vi "Write Source PDF File [ ].vi"(0 "PDF Report IN":refnum<class "PDF Report Class.lvclass">=refnum, 2 "TOC page":cluster{"Start":i32, "Number":i32}, 11 "error in (no error)":errorcluster, 13 "Last PageNumber":i32) -> (4 "PDF Report OUT":refnum<class "PDF Report Class.lvclass">, 15 "error out":errorcluster)   [LabVIEW 2020, in "Exaprom PDF.lvlib"]
doc: "Version 2.0\nDeveloped by Jean-Marc Simard\nCopyright © 2012, Exaprom Inc.\nAll rights reserved.\nLicense: BSD\n\nWith iTextSharp 4.1.6 (http://itextsharp.sourceforge.net)\nunder Mozilla Public License Version 1.1\n(http://www.mozilla.org/MPL/MPL-1.1.html)"
uses:
  <userlib>/labview-PDF-writer-master/Exaprom PDF.lvlib
  <userlib>/labview-PDF-writer-master/LV Class/PDF Report Class/PDF Report Class.lvclass
  <userlib>/labview-PDF-writer-master/LV Class/Fonts Class/Font Class.lvclass
  <userlib>/labview-PDF-writer-master/LV Class/Header and Footer Class/Header and Footer Class.lvclass
  <userlib>/labview-PDF-writer-master/Controls/Concatenate Controls/PDF File and position.ctl
  <userlib>/labview-PDF-writer-master/Controls/Concatenate Controls/PDF file source.ctl
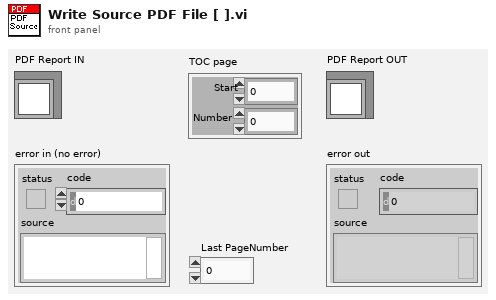
[diagram p1: front panel]
types:
  T1 = typedef "Exaprom PDF.lvlib/PDF File and position.ctl" = cluster{"Path":path, "Pages":string, "Source":T2, "Start at page old":i32, "Start at page new":i32, "Owner password":string}
  T2 = typedef "Exaprom PDF.lvlib/PDF file source.ctl" = enum16{"PDF Report", "File to add"}
  T3 = typedef "Exaprom PDF.lvlib/File Permission Parameters.ctl" = cluster{"User Password":string, "Owner Password":string, "Printing":enum16{"Allow Printing", "Allow Degraded Printing", "Don't Allow Printing"}, "Allow Modify Contents":bool, "Allow Copy":bool, "Allow Modify Annotations":bool, "Allow Fill In ":bool, "Allow Screen Readers":bool, "Allow Assembly":bool}
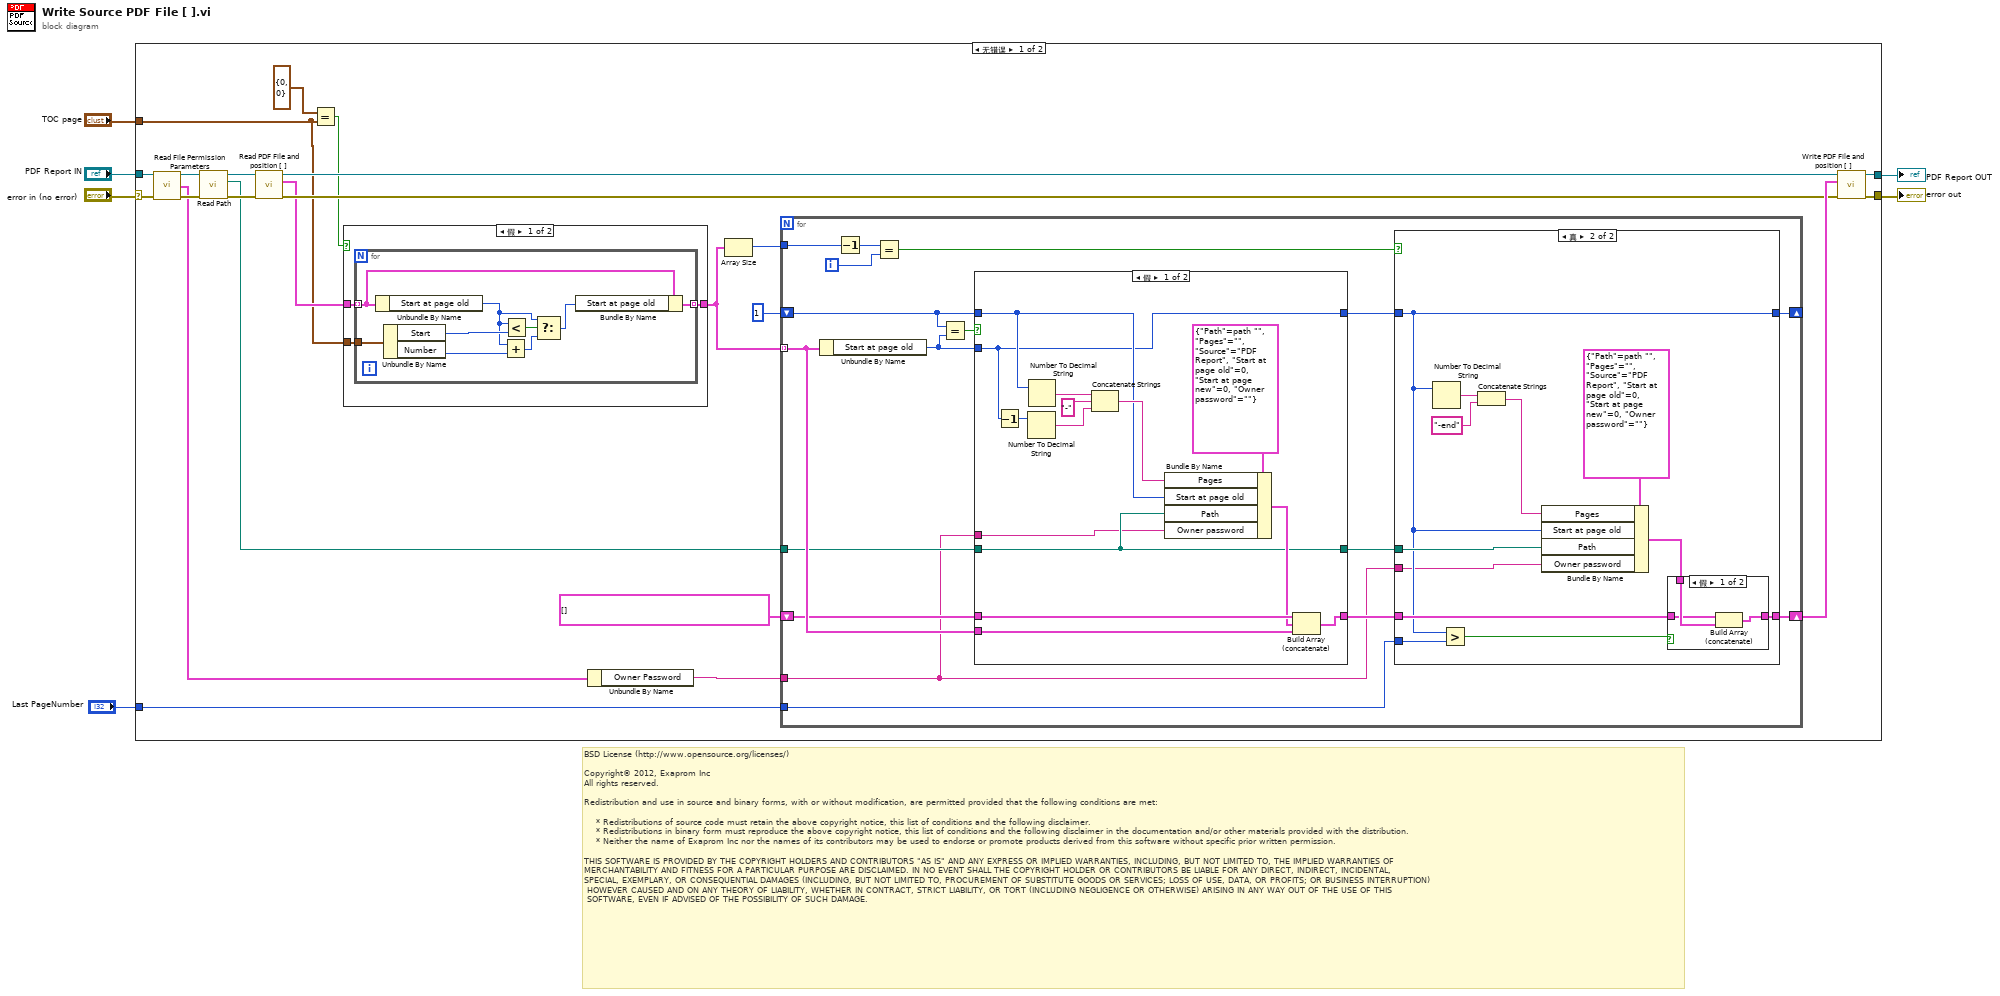
[diagram p0: block diagram]
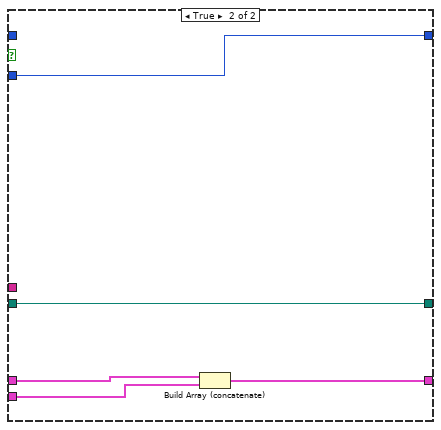
[diagram p5: hidden frame]
diagram:
  # "BSD License (http://www.opensource.org/licenses/)\n\nCopyright© 2012, Exaprom Inc\nAll rights reserved.\n\nRedistribution and use in source and binary forms, with or without modification, are permitted provided that the following conditions are met:\n\n    * Redistributions of source code must retain the above copyright notice, this list of conditions and the following disclaimer.\n    * Redistributions in binary form must reproduce the above copyright notice, this list of conditions and the following disclaimer in the documentation and/or other materials provided with the distribution.\n    * Neither the name of Exaprom Inc nor the names of its contributors may be used to endorse or promote products derived from this software without specific prior written permission.\n\nTHIS SOFTWARE IS PROVIDED BY THE COPYRIGHT HOLDERS AND CONTRIBUTORS \"AS IS\" AND ANY EXPRESS OR IMPLIED WARRANTIES, INCLUDING, BUT NOT LIMITED TO, THE IMPLIED WARRANTIES OF \nMERCHANTABILITY AND FITNESS FOR A PARTICULAR PURPOSE ARE DISCLAIMED. IN NO EVENT SHALL THE COPYRIGHT HOLDER OR CONTRIBUTORS BE LIABLE FOR ANY DIRECT, INDIRECT, INCIDENTAL,\nSPECIAL, EXEMPLARY, OR CONSEQUENTIAL DAMAGES (INCLUDING, BUT NOT LIMITED TO, PROCUREMENT OF SUBSTITUTE GOODS OR SERVICES; LOSS OF USE, DATA, OR PROFITS; OR BUSINESS INTERRUPTION)\n HOWEVER CAUSED AND ON ANY THEORY OF LIABILITY, WHETHER IN CONTRACT, STRICT LIABILITY, OR TORT (INCLUDING NEGLIGENCE OR OTHERWISE) ARISING IN ANY WAY OUT OF THE USE OF THIS\n SOFTWARE, EVEN IF ADVISED OF THE POSSIBILITY OF SUCH DAMAGE."
  n1 = case shown="无错误" "error in (no error)" {
    selector: "error in (no error)" -> [w15 w98]
    tunnel: "PDF Report IN" -> [w18 w97]
    tunnel: [w25 w97] -> w5
    tunnel: [w26 w98] -> w4
    tunnel: "Last PageNumber" -> [w17 _]
    tunnel: "TOC page" -> [w8 _]
    frame No Error {
      n2 = call-dynamic "Read File Permission Parameters.vi"("PDF Report Class in"=w18, "error in (no error)"=w15) -> ("PDF Report Class out"=w16:refnum<class "PDF Report Class.lvclass">, "File Permission Parameters"=w13:T3, "error out"=w14:errorcluster)  [unwired: 11 in]
      n3 = call-dynamic "Read Path.vi"("error in (no error)"=w14, "PDF Report Class in"=w16) -> ("error out"=w21:errorcluster, "Path"=w20:path, "PDF Report Class out"=w19:refnum<class "PDF Report Class.lvclass">)  [unwired: 7 in]
      n4 = call-dynamic "Read PDF File and position [ ].vi"("error in (no error)"=w21, "PDF Report Class in"=w19) -> ("error out"=w23:errorcluster, "PDF File and position [ ]"=w10:T1[], "PDF Report Class out"=w22:refnum<class "PDF Report Class.lvclass">)  [unwired: 7 in]
      n5 = Equal?(x=cluster{"Start":i32, "Number":i32} {"Start"=0, "Number"=0}, y=w8) -> (x = y?=w7:bool)
      n6 = case shown="假" w7 {
        tunnel: w10 -> [w32 w42]
        tunnel: [w31 w42] -> w9
        tunnel: w8 -> [w30 _]
        frame False {
          n7 = for {
            tunnel: w32 -> [w41] mode=indexing
            tunnel: [w40] -> w31 mode=indexing
            tunnel: w30 -> [w39]
            n8 = Unbundle By Name(w41) -> ("Start at page old"=w34:i32)
            n9 = Unbundle By Name(w39) -> ("Start"=w38:i32, "Number"=w33:i32)
            n10 = Add(x=w34, y=w33) -> (x+y=w35:i32)
            n11 = Less?(x=w34, y=w38) -> (x < y?=w37:bool)
            n12 = Select(t=w34, s=w37, f=w35) -> (s? t:f=w36:i32)
            n13 = Bundle By Name(cluster=w41, "Start at page old"=w36) -> (w40:T1)
          }
        }
        frame True {
        }
      }
      n14 = Unbundle By Name(w13) -> ("Owner Password"=w12:string)
      n15 = Array Size(array=w9) -> (size(s)=w27:i32)
      n16 = for {
        tunnel: w9 -> [w59] mode=indexing
        shift-right: [w50] -> _
        shift-left: 1 ("Start at page") -> [w48]
        shift-right: [w52] -> w24
        shift-left: T1[] [] -> [w57]
        tunnel: w27 -> [w56]
        tunnel: w20 -> [w46]
        tunnel: w17 -> [w44]
        tunnel: w12 -> [w43]
        i -> [w55]
        n17 = Unbundle By Name(w59) -> ("Start at page old"=w47:i32)
        n18 = Decrement(x=w56) -> (x-1=w54:i32)
        n19 = Equal?(x=w54, y=w55) -> (x = y?=w53:bool)
        n20 = Equal?(x=w48, y=w47) -> (x = y?=w58:bool)
        n21 = case shown="假" w58 {
          tunnel: [w80 w94] -> w49
          tunnel: w48 -> [w83 _]
          tunnel: w59 -> [w86 w95]
          tunnel: [w85 w96] -> w51
          tunnel: w57 -> [w87 w93]
          tunnel: w47 -> [w80 w94]
          tunnel: w46 -> [w79 w92]
          tunnel: [w79 w92] -> w45
          tunnel: w43 -> [w78 _]
          frame False {
            n22 = Decrement(x=w80) -> (x-1=w84:i32)
            n23 = Number To Decimal String(number=w84) -> (decimal integer string=w90:string)  [unwired: 1 in]
            n24 = Number To Decimal String(number=w83) -> (decimal integer string=w91:string)  [unwired: 1 in]
            n25 = Concatenate Strings(w91, "-" ("string"), w90) -> (w88:string)
            n26 = Bundle By Name(cluster=T1 {"Path"=path "", "Pages"="", "Source"=enum."PDF Report", "Start at page old"=0, "Start at page new"=0, "Owner password"=""} ("PDF File and position"), "Pages"=w88, "Start at page old"=w83, "Path"=w79, "Owner password"=w78) -> (w81:T1)
            n27 = Build Array (concatenate)(w87, w81, w86) -> (w85:T1[])
          }
          frame True {
            n28 = Build Array (concatenate)(w93, w95) -> (w96:T1[])
          }
        }
        n29 = case shown="真" w53 {
          tunnel: [w61 w67] -> w52
          tunnel: w51 -> [w61 w68]
          tunnel: [w60 w65] -> w50
          tunnel: w49 -> [w60 w65]
          tunnel: w45 -> [_ w66]
          tunnel: w44 -> [_ w64]
          tunnel: w43 -> [_ w62]
          frame False {
          }
          frame True {
            n30 = Number To Decimal String(number=w65) -> (decimal integer string=w73:string)  [unwired: 1 in]
            n31 = Greater?(x=w65, y=w64) -> (0:w63:bool)
            n32 = Concatenate Strings(w73, "-end" ("string")) -> (w71:string)
            n33 = Bundle By Name(cluster=T1 {"Path"=path "", "Pages"="", "Source"=enum."PDF Report", "Start at page old"=0, "Start at page new"=0, "Owner password"=""} ("PDF File and position"), "Pages"=w71, "Start at page old"=w65, "Path"=w66, "Owner password"=w62) -> (w69:T1)
            n34 = case shown="假" w63 {
              tunnel: w69 -> [w76 _]
              tunnel: w68 -> [w75 w77]
              tunnel: [w74 w77] -> w67
              frame False {
                n35 = Build Array (concatenate)(w75, w76) -> (w74:T1[])
              }
              frame True {
              }
            }
          }
        }
      }
      n36 = call-dynamic "Write PDF File and position [ ].vi"("error in (no error)"=w23, "PDF File and position [ ]"=w24, "PDF Report Class in"=w22) -> ("error out"=w26:errorcluster, "PDF Report Class out"=w25:refnum<class "PDF Report Class.lvclass">)  [unwired: 7 in]
    }
    frame Error {
    }
  }
  "PDF Report OUT" <- w5
  "error out" <- w4
